vi "MecanumDrive_Custom.vi"(6 "Rotation":dbl, 7 "Gyro Angle":dbl, 8 "error in (no error)":errorcluster, 9 "Y":dbl, 10 "X":dbl, 11 "RobotDriveDevRef":T1={"DevStatus"={"status"=FALSE, "code"=0, "source"=""}, "Motors[]"=[], "Square Inputs"=FALSE, "Max Output"=1.0}) -> (0 "error out":errorcluster, 2 "Motor Values":dbl[](array[numeric]), 3 "RobotDriveDevRef":T1={"DevStatus"={"status"=FALSE, "code"=0, "source"=""}, "Motors[]"=[], "Square Inputs"=FALSE, "Max Output"=1.0})   [LabVIEW 2014]
doc: "Configures the motors for holonomic driving. Holonomic driving allows you to move the robot in any direction without first rotating or maneuvering the robot.\n\nThis VI requires the robot to have either four omni-directional wheels and four motors mounted at 45 degree angles in the four corners of a square frame or to have four mecanum wheels driven by four motors.\n\nThe control input is intended to be connected directly to the X, Y, and Z axes of a joystick. The Y axis is inverted for you.\n\nThis software is licensed. Open the labview\\readme\\WPI Robotics Library Open Source License.txt file for more information."
uses:
  <vilib>/Rock Robotics/WPI/RobotDrive/WPI_RobotDriveDevRef.ctl
  <vilib>/Rock Robotics/WPI/MotorControl/WPI_MotorControlDeviceRef.ctl
  <vilib>/Rock Robotics/WPI/MotorControl/WPI_MotorControlType.ctl
  <vilib>/Rock Robotics/SystemInterfaces/Typedef/FPGA_TypedefDigitalModule.ctl
  <vilib>/Rock Robotics/SystemInterfaces/DIO/FPGA_DIOPWMChannel.ctl
  <vilib>/Rock Robotics/WPI/PWM/WPI_PWMDeadband.ctl
  <vilib>/Rock Robotics/WPI/CAN/Jaguar/SubVIs/WPI_CANJaguar_ControlMode.ctl
  <vilib>/Rock Robotics/WPI/CAN/TalonSRX/WPI_CANTalonSRX_APIControlMode.ctl
  <vilib>/Rock Robotics/WPI/PWM/WPI_PWMTransform_ConPane.ctl
  <vilib>/Rock Robotics/SystemInterfaces/NetworkCommunication/NetComm_UsageReport_ResourceType.ctl
  Robot Global Data.vi
  <vilib>/Rock Robotics/WPI/RobotDrive/WPI_RobotDriveSafetyCheck.vi
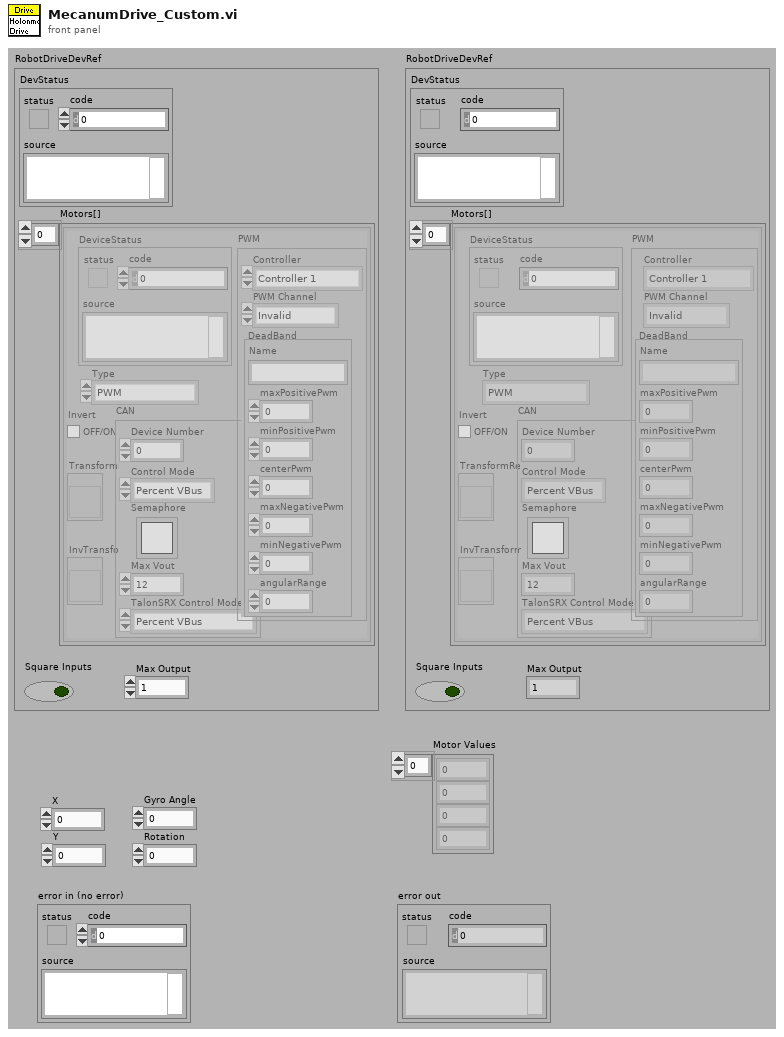
[diagram p1: front panel]
types:
  T1 = typedef "WPI_RobotDriveDevRef.ctl" = cluster{"DevStatus":errorcluster, "Motors[]":T2[], "Square Inputs":bool, "Max Output":dbl}
  T2 = typedef "WPI_MotorControlDeviceRef.ctl" = cluster{"DeviceStatus":errorcluster, "Type":T3, "PWM":cluster{"Controller":T4, "PWM Channel":T5, "DeadBand":T6}, "CAN":cluster{"Device Number":u8, "Control Mode":T7, "Semaphore":T8, "Max Vout":dbl, "TalonSRX Control Mode":T9}, "Invert":bool, "TransformRef":T10, "InvTransformRef":T10}
  T3 = typedef "WPI_MotorControlType.ctl" = enum16{"PWM", "CAN", "CANTalonSRX"}
  T4 = typedef "FPGA_TypedefDigitalModule.ctl" = enum16{"Controller 1"}
  T5 = typedef "FPGA_DIOPWMChannel.ctl" = enum8{"PWM 0", "PWM 1", "PWM 2", "PWM 3", "PWM 4", "PWM 5", "PWM 6", "PWM 7", "PWM 8", "PWM 9", "PWM MXP 0", "PWM MXP 1", "PWM MXP 2", "PWM MXP 3", "PWM MXP 4", "PWM MXP 5", "PWM MXP 6", "PWM MXP 7", "PWM MXP 8", "PWM MXP 9", "Invalid"}
  T6 = typedef "WPI_PWMDeadband.ctl" = cluster{"Name":string, "maxPositivePwm":i32, "minPositivePwm":i32, "centerPwm":i32, "maxNegativePwm":i32, "minNegativePwm":i32, "angularRange":u16}
  T7 = typedef "WPI_CANJaguar_ControlMode.ctl" = enum8{"Percent VBus", "Current", "Speed", "Position", "Voltage"}
  T8 = typedef "Semaphore RefNum" = refnum<k1>
  T9 = typedef "WPI_CANTalonSRX_APIControlMode.ctl" = enum8{"Percent VBus", "Speed", "Position", "Slave", "Unchanged / Invalid"}
  T10 = typedef "WPI_PWMTransform_ConPane.ctl" = refnum<vi>
  T11 = typedef "NetComm_UsageReport_ResourceType.ctl" = enum8{"Controller", "Module", "Language", "CANPlugin", "Accelerometer", "ADXL345", "AnalogChannel", "AnalogTrigger", "AnalogTriggerOutput", "CANJaguar", "Compressor", "Counter", "Dashboard", "DigitalInput", "DigitalOutput", "DriverStationCIO", "DriverStationEIO", "DriverStationLCD", "Encoder", "GearTooth", "Gyro", "I2C", "Framework", "Jaguar", "Joystick", "Kinect", "KinectStick", "PIDController", "Preferences", "PWM", "Relay", "RobotDrive", "SerialPort", "Servo", "Solenoid", "SPI", "Task", "Ultrasonic", "Victor", "Button", "Command", "AxisCamera", "PCVideoServer", "SmartDashboard", "Talon", "HiTechnicColorSensor", "HiTechnicAccel", "HiTechnicCompass", "SRF08", "AnalogOutput", "Victor SP", "Talon SRX", "CAN Talon SRX"}
  T12 = typedef "WPI_CANTalonSRX_GlobalStatus.ctl" = cluster{"Applied Throttle":dbl, "Module Enabled":bool, "CAN Error":errorcluster, "Closed Loop Error":dbl, "Forward Limit Switch Closed":bool, "Reverse Limit Switch Closed":bool, "Sensor Position":dbl, "Sensor Velocity":dbl, "Current":dbl, "Sticky Fault - Over Temp":bool, "Sticky Fault - Under Voltage":bool, "Sticky Fault - Forward Limit":bool, "Sticky Fault - Reverse Limit":bool, "Sticky Fault - Forward Soft Limit":bool, "Sticky Fault - Reverse Soft Limit":bool, "Brake is Enabled":bool, "Encoder Position":dbl, "Encoder Velocity":dbl, "Encoder Index Count":dbl, "Encoder A Pin State":bool, "Encoder B Pin State":bool, "Encoder Index Pin State":bool, "Analog In":dbl, "Analog In Velocity":dbl, "Temperature (C)":dbl, "Battery Voltage":dbl}
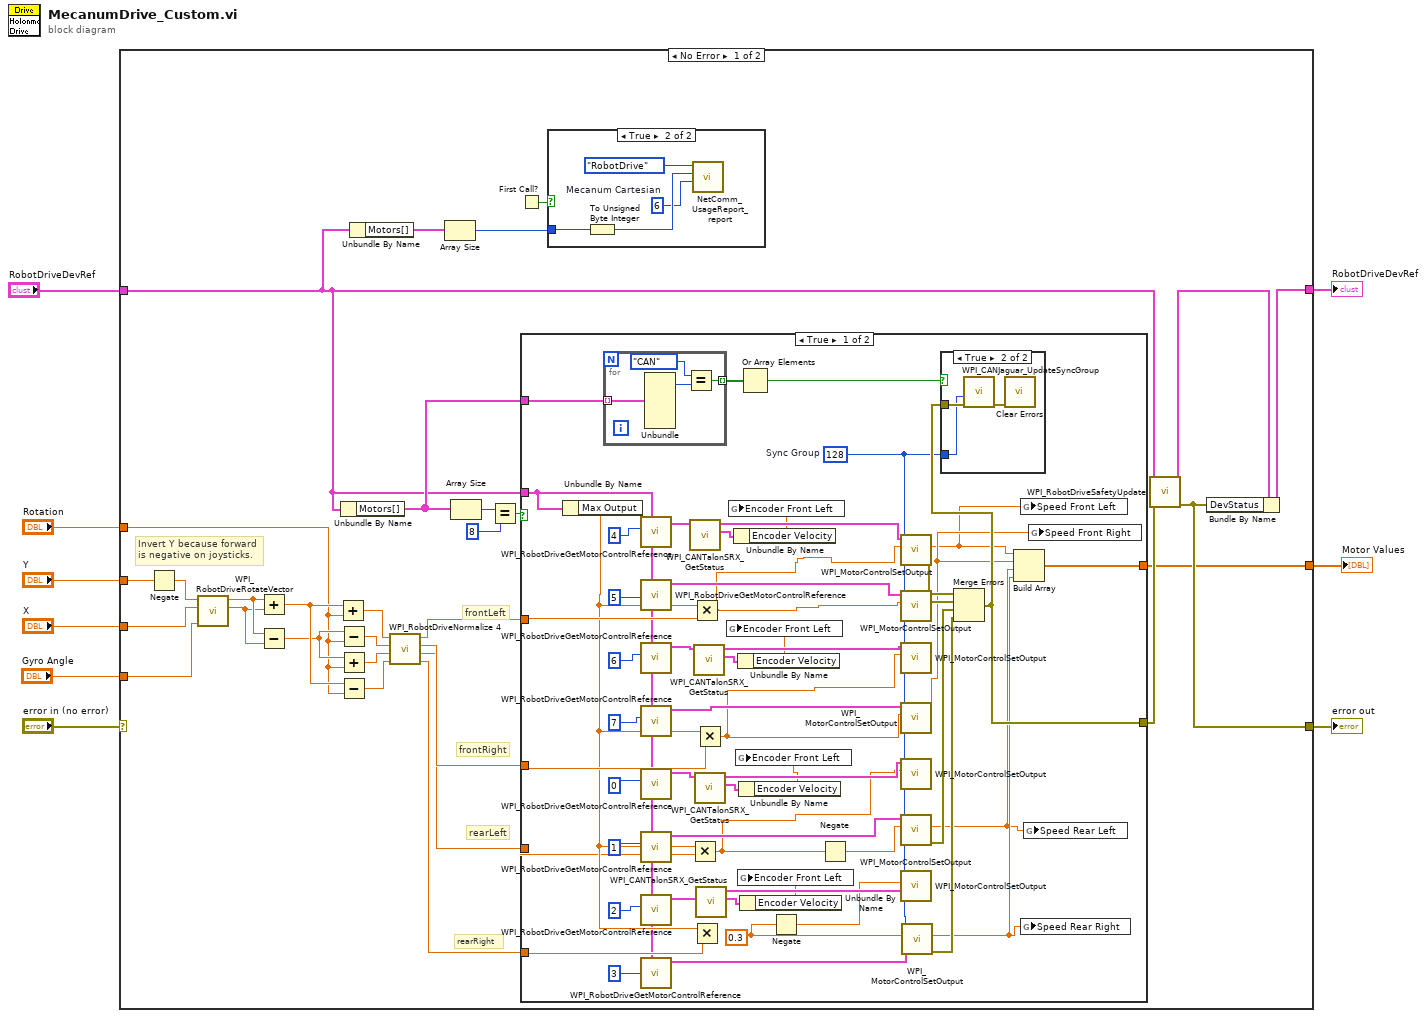
[diagram p0: block diagram]
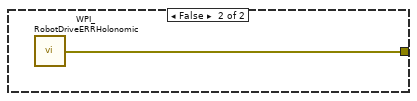
[diagram p4: hidden frame]
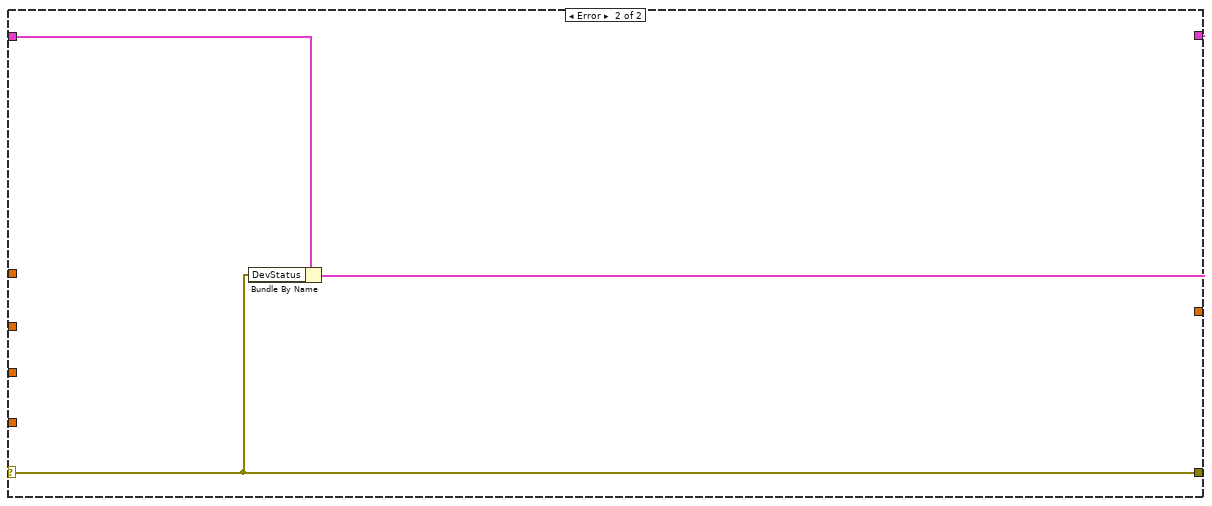
[diagram p5: hidden frame]
diagram:
  n1 = case shown="No Error" "error in (no error)" {
    selector: "error in (no error)" -> [_ w106]
    tunnel: "Y" -> [w21 _]
    tunnel: "X" -> [w26 _]
    tunnel: "RobotDriveDevRef" -> [w10 w108]
    tunnel: [w36 w107] -> w5
    tunnel: [w16 w106] -> w4
    tunnel: "Rotation" -> [w27 _]
    tunnel: "Gyro Angle" -> [w20 _]
    tunnel: [w14 _] -> w1
    frame No Error {
      # "Invert Y because forward is negative on joysticks."
      # "rearLeft"
      # "frontRight"
      # "rearRight"
      # "frontLeft"
      n2 = Negate(x=w21) -> (-x=w19:dbl)
      n3 = call <vilib>:"WPI_RobotDriveRotateVector.vi"("Angle"=w20, "X"=w26, "Y"=w19) -> ("X'"=w34:dbl, "Y'"=w35:dbl)  [unwired: 7 out]
      n4 = Add(x=w35, y=w34) -> (x+y=w32:dbl)
      n5 = Subtract(x=w35, y=w34) -> (x-y=w30:dbl)
      n6 = Add(x=w32, y=w27) -> (x+y=w28:dbl)
      n7 = Subtract(x=w30, y=w27) -> (x-y=w29:dbl)
      n8 = Add(x=w30, y=w27) -> (x+y=w31:dbl)
      n9 = Subtract(x=w32, y=w27) -> (x-y=w33:dbl)
      n10 = Unbundle By Name(w10) -> ("Motors[]"=w15:T2[])
      n11 = Unbundle By Name(w10) -> ("Motors[]"=w12:T2[])
      n12 = call <vilib>:"WPI_RobotDriveNormalize 4.vi"("D"=w33, "C"=w31, "B"=w29, "A"=w28) -> ("D'"=w23:dbl, "C'"=w22:dbl, "B'"=w24:dbl, "A'"=w25:dbl)
      n13 = Array Size(array=w12) -> (size(s)=w13:i32)
      n14 = Array Size(array=w15) -> (size(s)=w39:i32)
      n15 = Equal?(x=w39, y=8) -> (x = y?=w37:bool)
      n16 = First Call?() -> (First Call?: T/F=w11:bool)
      n17 = case shown="True" w37 {
        tunnel: w25 -> [w97 _]
        tunnel: w24 -> [w96 _]
        tunnel: w10 -> [w76 _]
        tunnel: [w84 w105] -> w18
        tunnel: w22 -> [w44 _]
        tunnel: w23 -> [w92 _]
        tunnel: w15 -> [w85 _]
        tunnel: [w83 _] -> w14
        frame True {
          w45 = 0.3
          w73 = u8 128  # Sync Group
          n18 = Unbundle By Name(w76) -> ("Max Output"=w91:dbl)
          n19 = for {
            tunnel: w85 -> [w101] mode=indexing
            tunnel: [w98] -> w86 mode=indexing
            n20 = Unbundle(w101) -> ("Type"=w100:T3)  [unwired: 6 out]
            n21 = Equal?(x=enum16{"PWM", "CAN"}."CAN" ("Type"), y=w100) -> (x = y?=w98:bool)
          }
          n22 = call <vilib>:"WPI_RobotDriveGetMotorControlReference.vi"("MotorIndex"=4, "RobotDriveDevRef"=w76) -> ("MotorControlDeviceRef"=w71:T2)  [unwired: 9 out]
          n23 = call <vilib>:"WPI_RobotDriveGetMotorControlReference.vi"("MotorIndex"=5, "RobotDriveDevRef"=w76) -> ("MotorControlDeviceRef"=w72:T2)  [unwired: 9 out]
          n24 = call <vilib>:"WPI_RobotDriveGetMotorControlReference.vi"("MotorIndex"=6, "RobotDriveDevRef"=w76) -> ("MotorControlDeviceRef"=w67:T2)  [unwired: 9 out]
          n25 = call <vilib>:"WPI_RobotDriveGetMotorControlReference.vi"("MotorIndex"=7, "RobotDriveDevRef"=w76) -> ("MotorControlDeviceRef"=w94:T2)  [unwired: 9 out]
          n26 = call <vilib>:"WPI_RobotDriveGetMotorControlReference.vi"("MotorIndex"=0, "RobotDriveDevRef"=w76) -> ("MotorControlDeviceRef"=w64:T2)  [unwired: 9 out]
          n27 = call <vilib>:"WPI_RobotDriveGetMotorControlReference.vi"("MotorIndex"=1, "RobotDriveDevRef"=w76) -> ("MotorControlDeviceRef"=w95:T2)  [unwired: 9 out]
          n28 = call <vilib>:"WPI_RobotDriveGetMotorControlReference.vi"("MotorIndex"=2, "RobotDriveDevRef"=w76) -> ("MotorControlDeviceRef"=w61:T2)  [unwired: 9 out]
          n29 = call <vilib>:"WPI_RobotDriveGetMotorControlReference.vi"("MotorIndex"=3, "RobotDriveDevRef"=w76) -> ("MotorControlDeviceRef"=w93:T2)  [unwired: 9 out]
          n30 = call <vilib>:"WPI_CANTalonSRX_GetStatus.vi"("CAN Talon SRX Ref"=w71) -> ("Talon SRX Status"=w69:T12, "CAN Talon SRX Ref Out"=w70:T2)  [unwired: 8 in, 1 out]
          n31 = Multiply(x=w91, y=w44) -> (x*y=w48:dbl)
          n32 = Multiply(x=w91, y=w97) -> (x*y=w49:dbl)
          n33 = Multiply(x=w91, y=w92) -> ()  [unwired: 1 out]
          n34 = call <vilib>:"WPI_CANTalonSRX_GetStatus.vi"("CAN Talon SRX Ref"=w67) -> ("Talon SRX Status"=w68:T12, "CAN Talon SRX Ref Out"=w66:T2)  [unwired: 8 in, 1 out]
          n35 = Multiply(x=w91, y=w96) -> (x*y=w50:dbl)
          n36 = call <vilib>:"WPI_CANTalonSRX_GetStatus.vi"("CAN Talon SRX Ref"=w64) -> ("Talon SRX Status"=w65:T12, "CAN Talon SRX Ref Out"=w63:T2)  [unwired: 8 in, 1 out]
          n37 = call <vilib>:"WPI_CANTalonSRX_GetStatus.vi"("CAN Talon SRX Ref"=w61) -> ("Talon SRX Status"=w62:T12, "CAN Talon SRX Ref Out"=w60:T2)  [unwired: 8 in, 1 out]
          n38 = Unbundle By Name(w69) -> ("Encoder Velocity"=w59:dbl)
          n39 = global write "Robot Global Data.vi" "Encoder Front Left"(w59) -> ()
          n40 = Unbundle By Name(w68) -> ("Encoder Velocity"=w58:dbl)
          n41 = global write "Robot Global Data.vi" "Encoder Front Left"(w58) -> ()
          n42 = Unbundle By Name(w65) -> ("Encoder Velocity"=w57:dbl)
          n43 = global write "Robot Global Data.vi" "Encoder Front Left"(w57) -> ()
          n44 = Or Array Elements(Boolean array=w86) -> (logical OR=w87:bool)
          n45 = Unbundle By Name(w62) -> ("Encoder Velocity"=w56:dbl)
          n46 = global write "Robot Global Data.vi" "Encoder Front Left"(w56) -> ()
          n47 = Negate(x=w45) -> (-x=w46:dbl)
          n48 = Negate(x=w48) -> (-x=w47:dbl)
          n49 = call <vilib>:"WPI_MotorControlSetOutput.vi"("Sync Group / Parameter Slot"=w73, "Output"=w49, "MotorControlDevRef"=w70) -> ("error out"=w88:errorcluster, "Motor Output"=w51:dbl)  [unwired: 2 in, 5 out]
          n50 = call <vilib>:"WPI_MotorControlSetOutput.vi"("Sync Group / Parameter Slot"=w73, "Output"=w49, "MotorControlDevRef"=w72) -> ("error out"=w55:errorcluster)  [unwired: 2 in, 6 out]
          n51 = call <vilib>:"WPI_MotorControlSetOutput.vi"("Sync Group / Parameter Slot"=w73, "Output"=w50, "MotorControlDevRef"=w66) -> ()  [unwired: 2 in, 7 out]
          n52 = call <vilib>:"WPI_MotorControlSetOutput.vi"("Sync Group / Parameter Slot"=w73, "Output"=w50, "MotorControlDevRef"=w94) -> ("Motor Output"=w52:dbl)  [unwired: 2 in, 6 out]
          n53 = call <vilib>:"WPI_MotorControlSetOutput.vi"("Sync Group / Parameter Slot"=w73, "Output"=w48, "MotorControlDevRef"=w63) -> ()  [unwired: 2 in, 7 out]
          n54 = call <vilib>:"WPI_MotorControlSetOutput.vi"("Sync Group / Parameter Slot"=w73, "Output"=w47, "MotorControlDevRef"=w95) -> ("error out"=w89:errorcluster, "Motor Output"=w53:dbl)  [unwired: 2 in, 5 out]
          n55 = call <vilib>:"WPI_MotorControlSetOutput.vi"("Sync Group / Parameter Slot"=w73, "Output"=w46, "MotorControlDevRef"=w60) -> ()  [unwired: 2 in, 7 out]
          n56 = call <vilib>:"WPI_MotorControlSetOutput.vi"("Sync Group / Parameter Slot"=w73, "Output"=w45, "MotorControlDevRef"=w93) -> ("error out"=w90:errorcluster, "Motor Output"=w54:dbl)  [unwired: 2 in, 5 out]
          n57 = Merge Errors(w88, w55, w89, w90) -> (w84:errorcluster)
          n58 = case shown="True" w87 {
            tunnel: w84 -> [_ w103]
            tunnel: w73 -> [_ w102]
            frame False {
            }
            frame True {
              n59 = call <vilib>:"WPI_CANJaguar_UpdateSyncGroup.vi"("error in (no error)"=w103, "Sync Group"=w102) -> ("error out"=w104:errorcluster)  [unwired: 9 out]
              n60 = call <vilib>:"Clear Errors.vi"("error in (no error)"=w104) -> ()  [unwired: 1 in, 6 out]
            }
          }
          n61 = Build Array(w51, w52, w53, w54) -> (w83:dbl[])
          n62 = global write "Robot Global Data.vi" "Speed Front Left"(w51) -> ()
          n63 = global write "Robot Global Data.vi" "Speed Rear Right"(w54) -> ()
          n64 = global write "Robot Global Data.vi" "Speed Rear Left"(w53) -> ()
          n65 = global write "Robot Global Data.vi" "Speed Front Right"(w52) -> ()
        }
        frame False {
          n66 = call <vilib>:"WPI_RobotDriveERRHolonomic.vi"() -> ("error out"=w105:errorcluster)
        }
      }
      n67 = case shown="True" w11 {
        tunnel: w13 -> [_ w42]
        frame False {
        }
        frame True {
          w40 = u8 6  # Mecanum Cartesian
          n68 = To Unsigned Byte Integer(number=w42) -> (unsigned 8bit integer=w41:u8)
          n69 = call <vilib>:"NetComm_UsageReport_report.vi"("Context"=w40, "Instance Number"=w41, "Resource Type"=NetComm_UsageReport_ResourceType."RobotDrive") -> ()  [unwired: 9 in]
        }
      }
      n70 = call <vilib>:"WPI_RobotDriveSafetyUpdate.vi"("error in (no error)"=w18, "RobotDriveDevRef"=w10) -> ("error out"=w16:errorcluster, "RobotDriveDevRef"=w17:T1)  [unwired: 8 out]
      n71 = Bundle By Name(cluster=w17, "DevStatus"=w16) -> (w36:T1)
    }
    frame Error {
      n72 = Bundle By Name(cluster=w108, "DevStatus"=w106) -> (w107:T1)
    }
  }
  "error out" <- w4
  "RobotDriveDevRef" <- w5
  "Motor Values" <- w1
